vi "saveTestParameters.vi"(8 "error in (no error)":errorcluster, 11 "Logger in":refnum<class "TestDataLog.lvclass">) -> (0 "error out":errorcluster, 3 "Logger out":refnum<class "TestDataLog.lvclass">)   [LabVIEW 2015, in "TestDataLog.lvclass"]
uses:
  TestDataLog.lvclass
  <userlib>/Common/Log/Log/Log.lvclass/Log.ctl
  TestDataLog.lvclass/TestDataLog.ctl
  <userlib>/Common/Log/Log/Log.lvclass
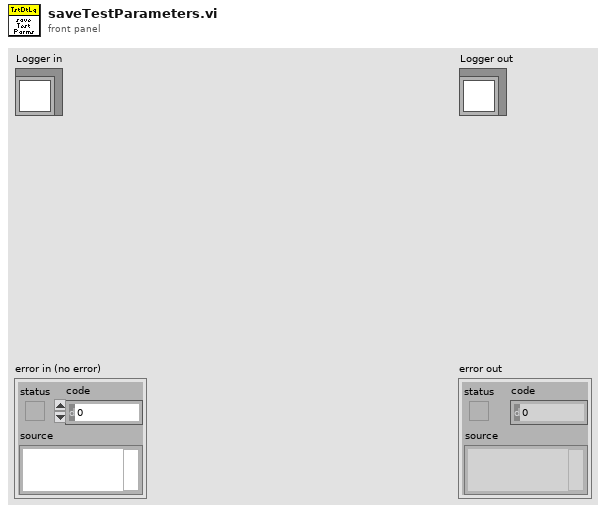
[diagram p1: front panel]
types:
  T1 = typedef "Preconditioning.ctl" = cluster{"Number of Preconditioning Cycles":u32}
  T2 = typedef "SystemController.ctl" = cluster{"PreconditioningRamp Rate (%/s)":dbl[unit], "Stiffness Test Ramp Rate (%/s)":dbl[unit], "Preconditioning Ramp Target":cluster{"Displacement":dbl[unit]}, "Stiffness Test Ramp Targets":cluster{"Displacement":dbl[unit], "Target Force":dbl[unit]}, "Settling":cluster{"Displacement Max StDev":dbl[unit], "Evaluation Time":dbl[unit]}}
  T3 = typedef "Log.lvlib/Log.ctl" = cluster{"Log Directory":path, "Log Filename Base":string, "Max records per file":u32, "Comment":string, "DUT ID":string}
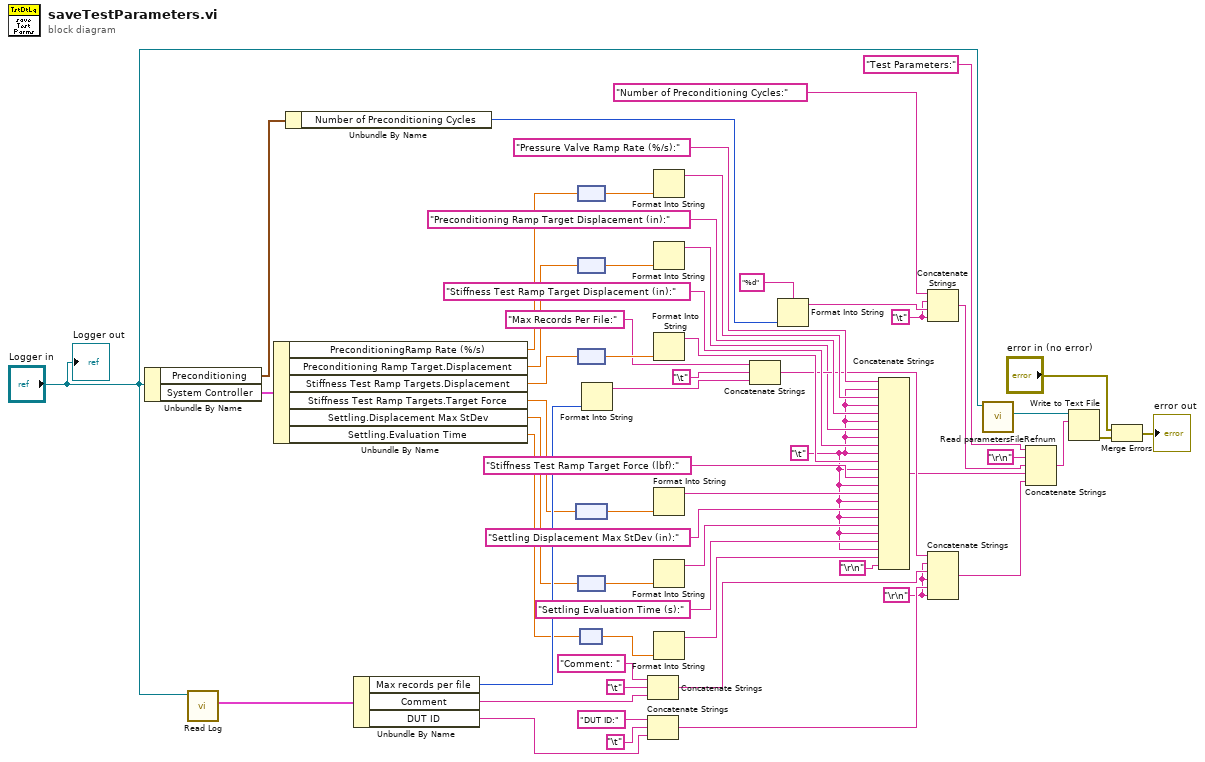
[diagram p0: block diagram]
diagram:
  w7 = "\r\n"
  w2 = "\t"
  w4 = "\t"
  n1 = Unbundle By Name("Logger in") -> ("Preconditioning"=w45:T1, "System Controller"=w40:T2)
  n2 = call <userlib>:"Read Log.vi"("Log in"="Logger in") -> ("Log"=w59:T3)  [unwired: 9 in, 1 out]
  n3 = Unbundle By Name(w40) -> ("PreconditioningRamp Rate (%/s)"=w38:dbl[unit], "Preconditioning Ramp Target.Displacement"=w32:dbl[unit], "Stiffness Test Ramp Targets.Displacement"=w28:dbl[unit], "Stiffness Test Ramp Targets.Target Force"=w26:dbl[unit], "Settling.Displacement Max StDev"=w21:dbl[unit], "Settling.Evaluation Time"=w17:dbl[unit])
  n4 = Unbundle By Name(w45) -> ("Number of Preconditioning Cycles"=w44:u32)
  n5 = Unbundle By Name(w59) -> ("Max records per file"=w58:u32, "Comment"=w52:string, "DUT ID"=w9:string)
  n6 = node(w26) -> (w27:dbl)
  n7 = node(w38) -> (w37:dbl)
  n8 = node(w32) -> (w33:dbl)
  n9 = node(w28) -> (w31:dbl)
  n10 = node(w21) -> (w23:dbl)
  n11 = node(w17) -> (w18:dbl)
  n12 = Format Into String(w58) -> (resulting string=w54:string)  [unwired: 3 in, 1 out]
  n13 = Concatenate Strings("Comment: " ("element"), "\t", w52) -> (w12:string)
  n14 = Concatenate Strings("DUT ID:" ("element"), "\t", w9) -> (w8:string)
  n15 = Format Into String(w37) -> (resulting string=w35:string)  [unwired: 3 in, 1 out]
  n16 = Format Into String(w33) -> (resulting string=w3:string)  [unwired: 3 in, 1 out]
  n17 = Format Into String(w31) -> (resulting string=w29:string)  [unwired: 3 in, 1 out]
  n18 = Format Into String(w27) -> (resulting string=w24:string)  [unwired: 3 in, 1 out]
  n19 = Format Into String(w23) -> (resulting string=w20:string)  [unwired: 3 in, 1 out]
  n20 = Format Into String(w18) -> (resulting string=w16:string)  [unwired: 3 in, 1 out]
  n21 = Concatenate Strings("Max Records Per File:" ("element"), "\t", w54) -> (w13:string)
  n22 = Format Into String(format string="%d", w44) -> (resulting string=w42:string)  [unwired: 2 in, 1 out]
  n23 = Concatenate Strings("Pressure Valve Ramp Rate (%/s):", w2, w35, w2, "Preconditioning Ramp Target Displacement (in):", w2, w3, w2, "Stiffness Test Ramp Target Displacement (in):", w2, w29, w2, "Stiffness Test Ramp Target Force (lbf):", w2, w24, w2, "Settling Displacement Max StDev (in):", w2, w20, w2, "Settling Evaluation Time (s):", w2, w16, "\r\n") -> (w6:string)
  n24 = Concatenate Strings("Number of Preconditioning Cycles:", w4, w42, w4) -> (w41:string)
  n25 = Concatenate Strings(w13, w7, w12, w7, w8, w7) -> (w5:string)
  n26 = call <userlib>:"Read parametersFileRefnum.vi"("Log in"="Logger in") -> ("parametersFileRefnum"=w51:refnum<file>)  [unwired: 9 in, 1 out]
  n27 = Concatenate Strings("Test Parameters:", "\r\n", w41, w6, w5) -> (w50:string)
  n28 = Write to Text File(file (use dialog)=w51, text=w50) -> (error out=w48:errorcluster)  [unwired: 2 in, 2 out]
  n29 = Merge Errors("error in (no error)", w48) -> (→"error out":errorcluster)
  "Logger out" <- "Logger in"
